vi "HAL & MATH Test (SubVI).vi"(11 "Notifier in":refnum<notifier>) -> ()   [LabVIEW 2014]
uses:
  MATH/MathLoop/TypeDefs/ParsedExpression.ctl
  MATH/MathLoop/TypeDefs/typeMed.ctl
  MATH/MathLoop/TypeDefs/Conf. Gral.ctl
  MATH/MathLoop/MathLoop.lvlib
panel:
  in  "stop 2":bool
  in  "Array 2":sgl[](array[slide]) scale=-10.0..10.0
  in  "Array":T1[](array[typedef])
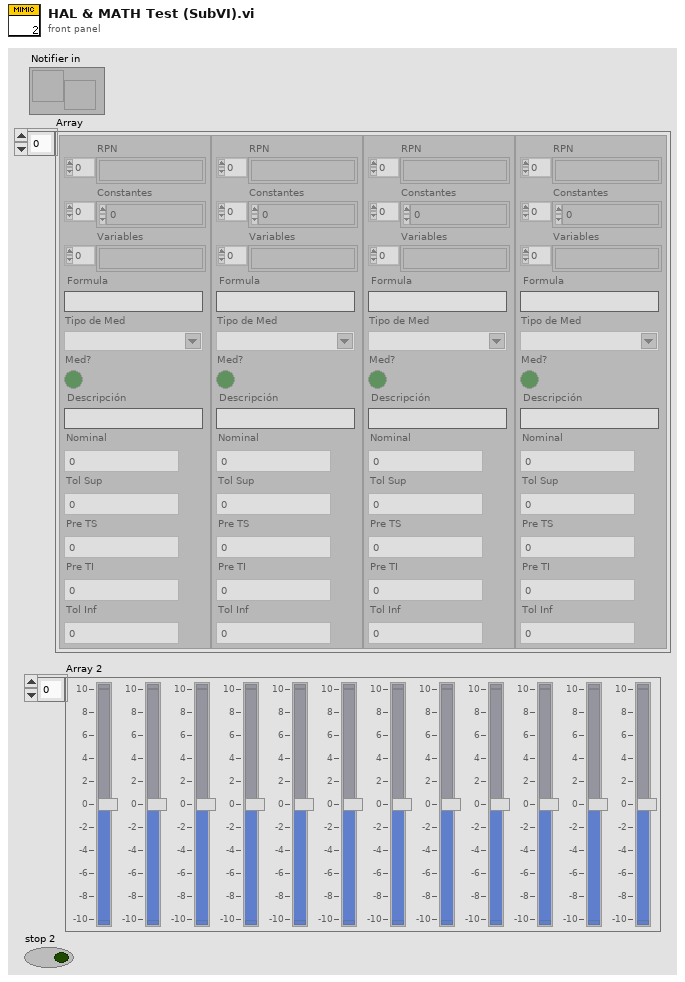
[diagram p1: front panel]
types:
  T1 = typedef "MathLoop.lvlib/ParsedExpression.ctl" = cluster{"RPN ":string[], "Constantes":sgl[], "Variables":string[], "Formula":string, "Tipo de Med":T2, "Med?":bool, "Descripción":string, "Nominal":sgl, "Tol Sup":sgl, "Pre TS":sgl, "Pre TI":sgl, "Tol Inf":sgl}
  T2 = typedef "MathLoop.lvlib/typeMed.ctl" = string
  T3 = typedef "MathLoop.lvlib/Conf. Gral.ctl" = cluster{"Engranometro":cluster{"Cant. Dientes x pieza":i32, "Nro. Dientes (Frp)":i32, "Armonicas":i32}}
  T4 = cluster{"Kcte":sgl[], "Dcte":sgl[], "Aux":sgl[][], "Transductores":sgl[][]}
  T5 = cluster{"Variable Data Out":cluster{"Kcte":sgl[], "Dcte":sgl[], "Aux":sgl[][], "Transductores":sgl[][]}, "Array":sgl[], T1[], "Array Med":sgl[][], "Conf. General":T3}
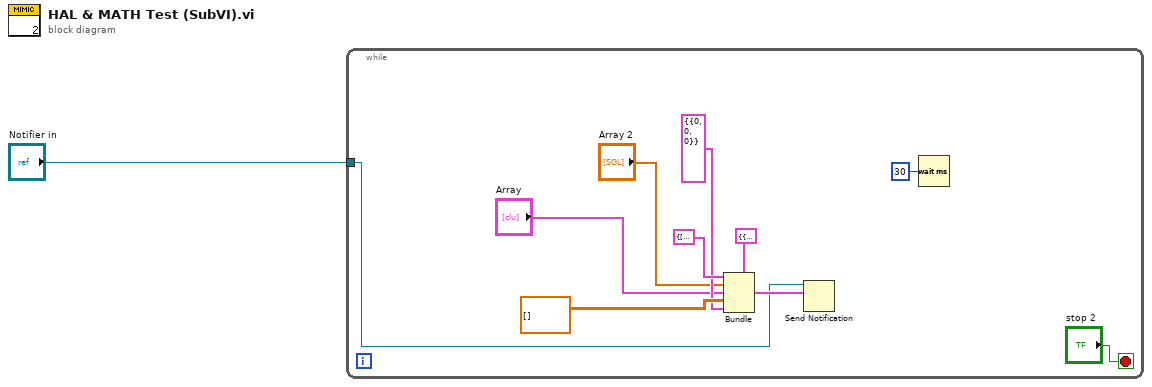
[diagram p0: block diagram]
diagram:
  n1 = while {
    tunnel: "Notifier in" -> [w6]
    stop <- "stop 2" stop-if-true
    n2 = Bundle(cluster=T5 {"Variable Data Out"={"Kcte"=[], "Dcte"=[], "Aux"=[], "Transductores"=[]}, "Array"=[], [], "Array Med"=[], "Conf. General"={"Engranometro"={"Cant. Dientes x pieza"=0, "Nro. Dientes (Frp)"=0, "Armonicas"=0}}} ("output cluster"), "Variable Data Out"=T4 {"Kcte"=[], "Dcte"=[], "Aux"=[], "Transductores"=[]}, "Array"="Array 2", "Array", "Array Med"=sgl[][] [], "Conf. General"=T3 {"Engranometro"={"Cant. Dientes x pieza"=0, "Nro. Dientes (Frp)"=0, "Armonicas"=0}}) -> (w11:T5)
    n3 = Send Notification(notification=w11, notifier=w6) -> ()  [unwired: 1 in, 2 out]
    n4 = Wait (ms)(milliseconds to wait=u32 30) -> ()  [unwired: 1 out]
  }
